vi "calc_conveyor.vi"(10 "Conveyor Command Inputs":T1, 11 "Conveyor Sensor Inputs":T2) -> (3 "Conveyor Outputs":T3={"Bottom Conveyor Speed"=0.5, "Top Conveyor Speed"=0.5, "Bottom Conveyor State"=enum."No Ball", "Top Conveyor State"=enum."Reset", "Accepting Balls"=FALSE, "Number of Balls"=0})   [LabVIEW 2012]
uses:
  Conveyor_outputs.ctl
  Conveyor module state.ctl
  Sensor_Input_Conveyor.ctl
  Input_Command_Conveyor.ctl
panel:
  in  "Load Speed":dbl=0.5
  in  "Adjust Speed":dbl=0.3
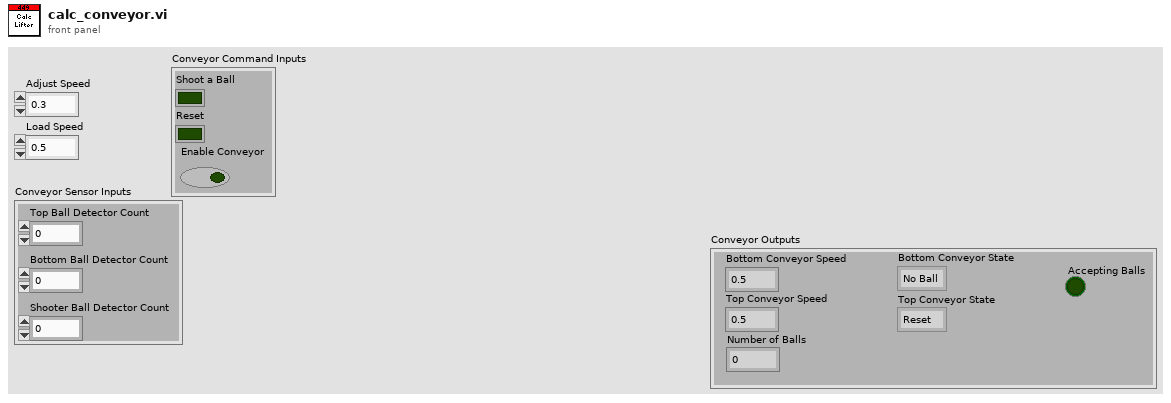
[diagram p1: front panel]
types:
  T1 = typedef "Input_Command_Conveyor.ctl" = cluster{"Shoot a Ball":bool, "Reset":bool, "Enable Conveyor":bool}
  T2 = typedef "Sensor_Input_Conveyor.ctl" = cluster{"Top Ball Detector Count":i32, "Bottom Ball Detector Count":i32, "Shooter Ball Detector Count":i32}
  T3 = typedef "Conveyor_outputs.ctl" = cluster{"Bottom Conveyor Speed":dbl, "Top Conveyor Speed":dbl, "Bottom Conveyor State":T4, "Top Conveyor State":T4, "Accepting Balls":bool, "Number of Balls":i32}
  T4 = typedef "Conveyor module state.ctl" = enum16{"No Ball", "Has Ball", "Ball Below Hold", "Ball Above Hold", "Outputting Ball", "Reset"}
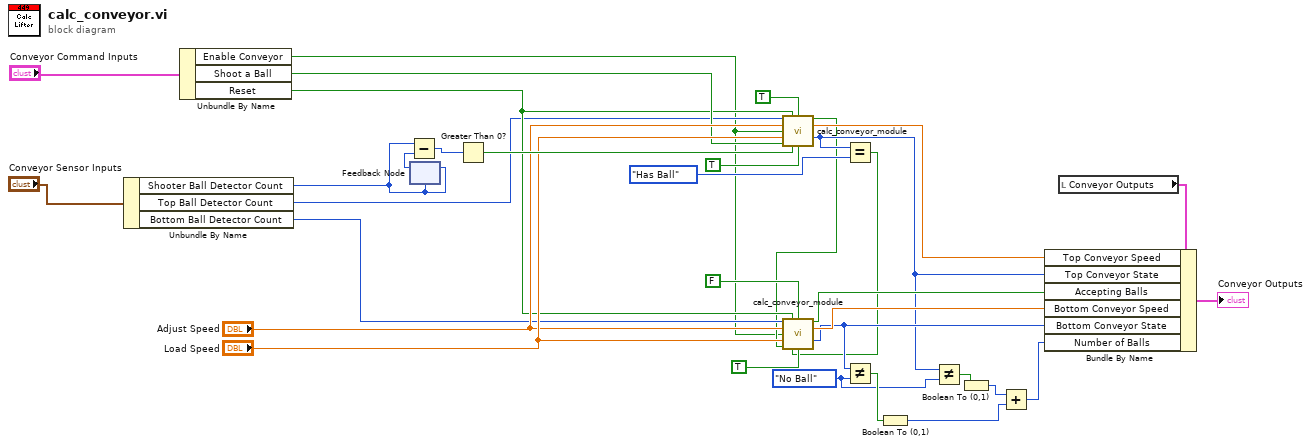
[diagram p0: block diagram]
diagram:
  w9 = Conveyor_module_state."No Ball" ("y")
  n1 = Unbundle By Name("Conveyor Sensor Inputs") -> ("Shooter Ball Detector Count"=w13:i32, "Top Ball Detector Count"=w12:i32, "Bottom Ball Detector Count"=w11:i32)
  n2 = Unbundle By Name("Conveyor Command Inputs") -> ("Enable Conveyor"=w1:bool, "Shoot a Ball"=w15:bool, "Reset"=w14:bool)
  n3 = feedback-in #1(w13) -> ()
  n4 = feedback #1(w13) -> (w32:i32)
  n5 = Subtract(x=w13, y=w32) -> (x-y=w31:i32)
  n6 = Greater Than 0?(x=w31) -> (x > 0?=w30:bool)
  n7 = call "calc_conveyor_module.vi"("Ball Detector Count"=w12, "Reset"=w14, "Is Top Module"=TRUE, "Adjust Speed"="Adjust Speed", "Enable Conveyor"=w1, "Load Speed"="Load Speed", "Push Ball Out"=w15, "Ball is out"=w30, "Accept Balls?"=TRUE) -> ("Accepting Balls"=w3:bool, "Conveyor Speed"=w25:dbl, "Lifter Module State"=w8:T4)  [unwired: 4 in]
  n8 = Equal?(x=w8, y=Conveyor_module_state."Has Ball" ("Lifter Module State")) -> (x = y?=w2:bool)
  n9 = call "calc_conveyor_module.vi"("Ball Detector Count"=w11, "Reset"=w14, "Is Top Module"=FALSE, "Adjust Speed"="Adjust Speed", "Enable Conveyor"=w1, "Load Speed"="Load Speed", "Push Ball Out"=w3, "Ball is out"=w2, "Accept Balls?"=TRUE) -> ("Accepting Balls"=w26:bool, "Conveyor Speed"=w27:dbl, "Lifter Module State"=w19:T4)  [unwired: 4 in]
  n10 = Not Equal?(x=w19, y=w9) -> (x != y?=w10:bool)
  n11 = Boolean To (0,1)(Boolean=w10) -> (0, 1=w5:i16)
  n12 = Not Equal?(x=w8, y=w9) -> (x != y?=w7:bool)
  n13 = Boolean To (0,1)(Boolean=w7) -> (0, 1=w6:i16)
  n14 = Add(x=w6, y=w5) -> (x+y=w4:i16)
  n15 = local read "Conveyor Outputs"() -> (w28:T3)
  n16 = Bundle By Name(cluster=w28, "Top Conveyor Speed"=w25, "Top Conveyor State"=w8, "Accepting Balls"=w26, "Bottom Conveyor Speed"=w27, "Bottom Conveyor State"=w19, "Number of Balls"=w4) -> (→"Conveyor Outputs":T3)
